vi "IR calculator.vi"(8 "Clear":i16, 9 "Blue":i16, 10 "Green":i16, 11 "Red":i16) -> (2 "IR":dbl)   [LabVIEW 2014, in "AMS TS3472 Light Sensor.lvlib" / "AMS TCS3472.lvclass"]
uses:
  AMS TCS3472.lvclass
panel:
  out "x-y":i16
  out "result":i16
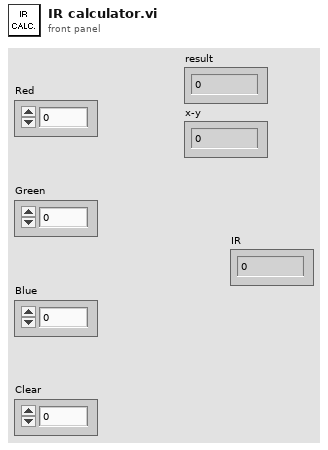
[diagram p1: front panel]
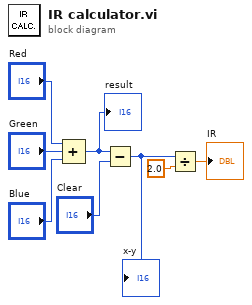
[diagram p0: block diagram]
diagram:
  n1 = Compound Arithmetic op=ADD("Red", "Green", "Blue") -> (w5:i16)
  "result" <- w5
  n2 = Subtract(x=w5, y="Clear") -> (x-y=w3:i16)
  "x-y" <- w3
  n3 = Divide(x=w3, y=2.0) -> (x/y=→"IR":dbl)
